vi "nirviAccSaturate.vi"(1 "y":i32, 2 "x":i32) -> (0 "x+y":i32)   [LabVIEW 2020]
doc: "Computes the sum of two 32-bit numbers using saturation arithmetic to avoid integer overflow by returning a maximum or minimum value."
uses:
  <vilib>/rvi/Arithmetic/AddSubMult/XNode/nirviSatArithmetic.xnode
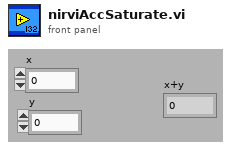
[diagram p1: front panel]
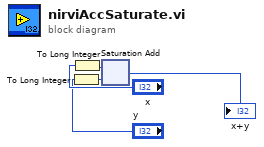
[diagram p0: block diagram]
diagram:
  n1 = To Long Integer(number="y") -> (32bit integer=w4:i32)
  n2 = To Long Integer(number="x") -> (32bit integer=w3:i32)
  n3 = xnode "Saturation Add"("x"=w3, "y"=w4) -> ("x+y"=→"x+y":i32)
